vi "Create Node.vi"(8 "error in (no error)":errorcluster, 10 "Type":T1, 11 "AST in":refnum<class "AST.lvclass">) -> (0 "error out":errorcluster, 2 "NodeRef":refnum<data-value>, 3 "AST out":refnum<class "AST.lvclass">)   [LabVIEW 2020, in "PicoG-ParserLexer.lvlib" / "AST.lvclass"]
doc: "Creates a new node with the specified type. The AST instance keeps track of all nodes created; any nodes not disposed of yet when an AST instance is cleaned up will be cleaned up.\n\n<b>Error Codes:</b>\n<b>1556</b>: AST instance invalid. AST instances must be initialized with Ctor"
uses:
  AST.lvclass
  Node/Node.lvclass
  AST Node Type.ctl
  PicoG-ParserLexer.lvlib
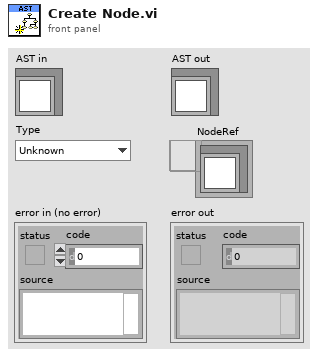
[diagram p1: front panel]
types:
  T1 = typedef "PicoG-ParserLexer.lvlib/AST Node Type.ctl" = enum16{"Unknown", "Keyword", "Array", "Cluster", "Numeric", "Boolean", "String", "Identifier"}
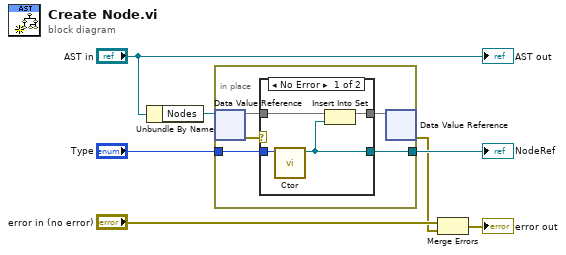
[diagram p0: block diagram]
diagram:
  n1 = Unbundle By Name("AST in") -> ("Nodes"=w5:refnum<data-value>)
  n2 = in-place {
    in-place-border: "Type" -> [w12]
    in-place-border: [w8] -> w3
    n3 = in-place-dvr #1(w5) -> (w10:set{refnum<data-value>}, w11:errorcluster)
    n4 = case shown="No Error" w11 {
      tunnel: w12 -> [w16 _]
      tunnel: w10 -> [w15 w17]
      tunnel: [w14 w17] -> w9
      tunnel: [w13 _] -> w8
      frame No Error {
        n5 = call "Ctor.vi"("Type"=w16) -> ("NodeRef"=w13:refnum<data-value>)  [unwired: 9 in, 1 out]
        n6 = Insert Into Set(10:w13, 11:w15) -> (3:w14:set{refnum<data-value>})  [unwired: 1 out]
      }
      frame Error {
      }
    }
    n7 = in-place-dvr #1(w9) -> (w1:errorcluster)  [unwired: 1 out]
  }
  "NodeRef" <- w3
  n8 = Merge Errors("error in (no error)", w1) -> (→"error out":errorcluster)
  "AST out" <- "AST in"
